vi "RSZVB Define Pulse Generator.vi"(0 "VISA session":refnum<visa-resource-name>, 1 "Single/Train Pulse Period (100.0e-6 s)":dbl=0.0001 format="%^.3e", 2 "Pulse Mode (0)":i32(ring) items=["Channel Specific", "Continuous Pulse"], 5 "Channel (1)":i32=1, 7 "Generator (1)":i32=1, 9 "Pulse Type (0)":i32(ring) items=["Single Pulse", "Pulse Train", "Constant High", "Constant Low"], 11 "error in (no error)":errorcluster {"code" format="%.0x"}, 12 "Pulse Polarity (0)":i32(ring) items=["Normal", "Inverted"], 13 "Pulse Width (0.5e-6 s)":dbl=5e-07 format="%^.3e") -> (4 "dup VISA session":refnum<visa-resource-name>, 15 "error out":errorcluster {"code" format="%.0x"})   [LabVIEW 2011]
doc: "This VI defines the properties of the pulse generator signals.\n\nNote(s):\n\n(1) This VI is available only with option R&S ZVA-K27.\n\nRemote-control command(s):\n[SENSe<Ch>:]PULSe:GENerator<gen_no>:TYPE SINGle | TRAin | CHIGh | CLOW\n[SENSe<Ch>:]PULSe:GENerator<gen_no>:WIDTh\n[SENSe<Ch>:]PULSe:GENerator<gen_no>:PERiod\n[SENSe<Ch>:]PULSe:GENerator<gen_no>:TRAin:PERiod\n[SENSe<Ch>:]PULSe:GENerator<gen_no>:POLarity NORMal | INVerted\n[SENSe<Ch>:]PULSe:GENerator<gen_no>:MODE CSPecific | CONTinuous"
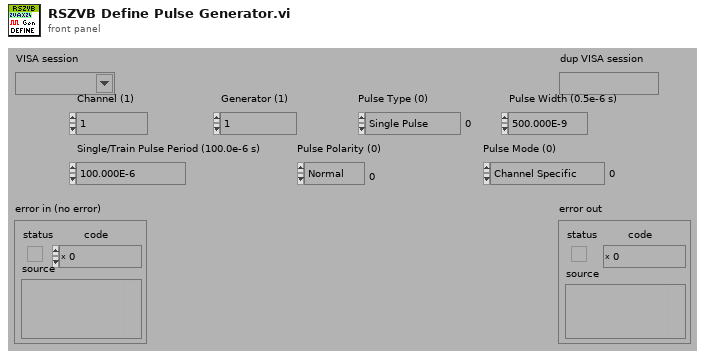
[diagram p1: front panel]
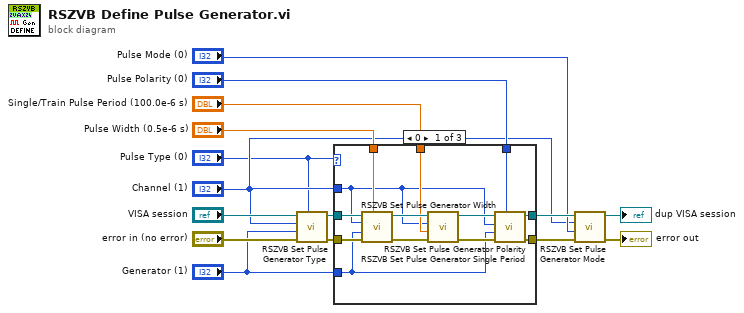
[diagram p0: block diagram]
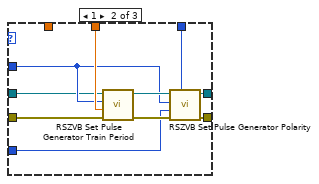
[diagram p2: hidden frame]
diagram:
  n1 = call "RSZVB Set Pulse Generator Type.vi"("Pulse Type (0)"="Pulse Type (0)", "error in (no error)"="error in (no error)", "Generator (1)"="Generator (1)", "Channel (1)"="Channel (1)", "VISA session"="VISA session") -> ("error out"=w10:errorcluster, "dup VISA session"=w11:refnum<visa-resource-name>)  [unwired: 5 in]
  n2 = case shown="0" "Pulse Type (0)" {
    tunnel: w11 -> [w28 w30 w40]
    tunnel: w10 -> [w27 w29 w39]
    tunnel: [w24 w37 w39] -> w9
    tunnel: [w21 w35 w40] -> w8
    tunnel: "Single/Train Pulse Period (100.0e-6 s)" -> [w20 w34 _]
    tunnel: "Pulse Width (0.5e-6 s)" -> [w19 _ _]
    tunnel: "Generator (1)" -> [w18 w33 _]
    tunnel: "Pulse Polarity (0)" -> [w17 w32 _]
    tunnel: "Channel (1)" -> [w16 w31 _]
    frame 0 {
      n3 = call "RSZVB Set Pulse Generator Width.vi"("Pulse Width (0.5e-6 s)"=w19, "error in (no error)"=w27, "Generator (1)"=w18, "Channel (1)"=w16, "VISA session"=w28) -> ("error out"=w26:errorcluster, "dup VISA session"=w23:refnum<visa-resource-name>)  [unwired: 5 in]
      n4 = call "RSZVB Set Pulse Generator Single Period.vi"("error in (no error)"=w26, "Single Pulse Period (100.0e-6 s)"=w20, "Channel (1)"=w16, "VISA session"=w23) -> ("error out"=w25:errorcluster, "dup VISA session"=w22:refnum<visa-resource-name>)  [unwired: 6 in]
      n5 = call "RSZVB Set Pulse Generator Polarity.vi"("Pulse Polarity (0)"=w17, "error in (no error)"=w25, "Generator (1)"=w18, "Channel (1)"=w16, "VISA session"=w22) -> ("error out"=w24:errorcluster, "dup VISA session"=w21:refnum<visa-resource-name>)  [unwired: 5 in]
    }
    frame 1 {
      n6 = call "RSZVB Set Pulse Generator Train Period.vi"("error in (no error)"=w29, "Train Pulse Period (100.0e-6 s)"=w34, "Channel (1)"=w31, "VISA session"=w30) -> ("error out"=w38:errorcluster, "dup VISA session"=w36:refnum<visa-resource-name>)  [unwired: 6 in]
      n7 = call "RSZVB Set Pulse Generator Polarity.vi"("Pulse Polarity (0)"=w32, "error in (no error)"=w38, "Generator (1)"=w33, "Channel (1)"=w31, "VISA session"=w36) -> ("error out"=w37:errorcluster, "dup VISA session"=w35:refnum<visa-resource-name>)  [unwired: 5 in]
    }
    frame Default {
    }
  }
  n8 = call "RSZVB Set Pulse Generator Mode.vi"("error in (no error)"=w9, "Pulse Mode (0)"="Pulse Mode (0)", "Channel (1)"="Channel (1)", "VISA session"=w8) -> ("error out"=→"error out":errorcluster, "dup VISA session"=→"dup VISA session":refnum<visa-resource-name>)  [unwired: 6 in]
